vi "Calculate time to acquire stack.vi"(8 "error in (no error)":errorcluster, 11 "Tomo in":refnum<class "Tomo.lvclass">) -> (0 "error out":errorcluster, 3 "Tomo out":refnum<class "Tomo.lvclass">)   [LabVIEW 2012, in "Tomo.lvclass"]
uses:
  Tomo.lvclass
  Tomo.lvclass/Tomo.ctl
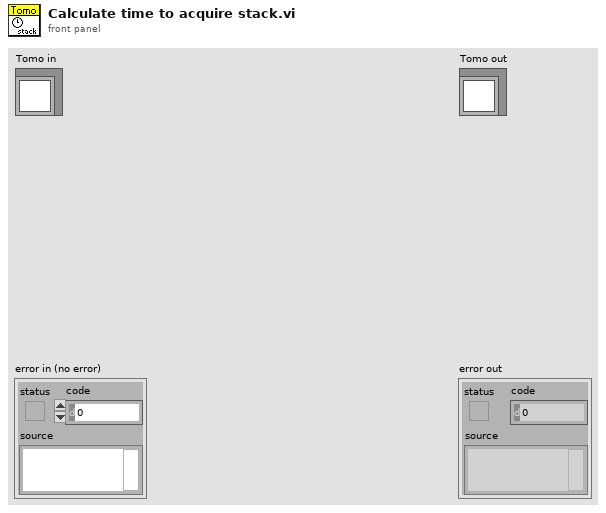
[diagram p1: front panel]
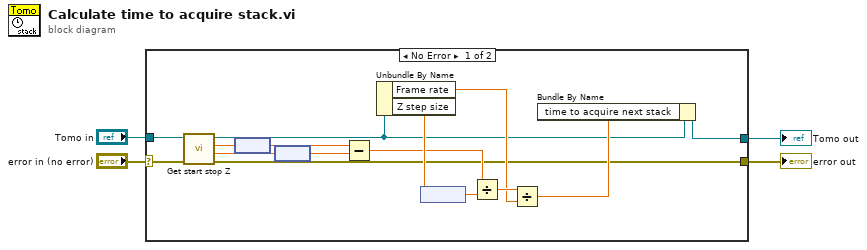
[diagram p0: block diagram]
diagram:
  n1 = case shown="No Error" "error in (no error)" {
    selector: "error in (no error)" -> [w17 w21]
    tunnel: [w9 w21] -> w3
    tunnel: [w13 w20] -> w1
    tunnel: "Tomo in" -> [w11 w20]
    frame No Error {
      n2 = call-dynamic "Get start stop Z.vi"("error in (no error)"=w17, "Tomo in"=w11) -> ("error out"=w9:errorcluster, "Z start"=w7:dbl[unit], "Z stop"=w8:dbl[unit], "Tomo out"=w10:refnum<class "Tomo.lvclass">)  [unwired: 4 in, 2 out]
      n3 = node(w8) -> (w6:dbl)
      n4 = node(w7) -> (w5:dbl)
      n5 = Subtract(x=w6, y=w5) -> (x-y=w16:dbl)
      n6 = Unbundle By Name(w10) -> ("Frame rate"=w14:dbl[unit], "Z step size"=w19:dbl[unit])
      n7 = node(w19) -> (w18:dbl)
      n8 = Divide(x=w16, y=w18) -> (x/y=w15:dbl)
      n9 = Divide(x=w15, y=w14) -> (x/y=w12:dbl[unit])
      n10 = Bundle By Name(cluster=w10, "time to acquire next stack"=w12) -> (w13:refnum<class "Tomo.lvclass">)
    }
    frame Error {
    }
  }
  "error out" <- w3
  "Tomo out" <- w1
